vi "SO55 Create Monitor Task.vi"(2 "error in":errorcluster, 3 "Input":T1) -> (0 "error out":errorcluster, 1 "task out":refnum<k21>)   [LabVIEW 2012]
uses:
  <vilib>/DAQmx/create/channels.llb/DAQmx Create Channel (AI-Voltage-Basic).vi
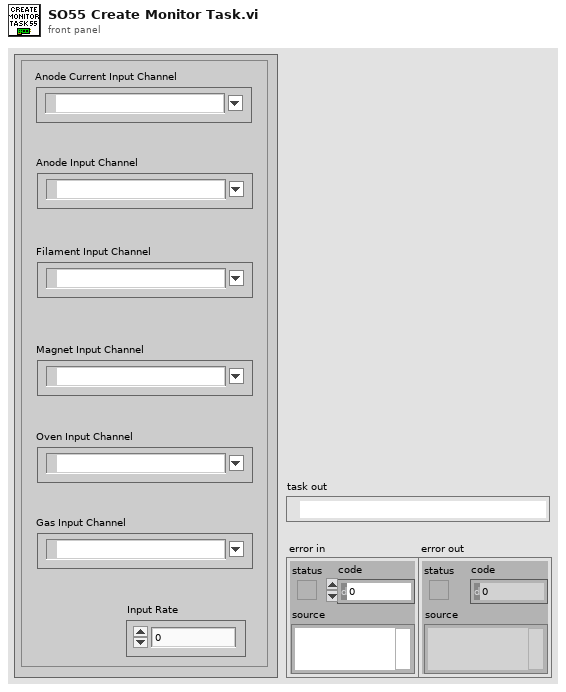
[diagram p1: front panel]
types:
  T1 = cluster{"Anode Input Channel":tag, "Filament Input Channel":tag, "Magnet Input Channel":tag, "Oven Input Channel":tag, "Gas Input Channel":tag, "Input Rate":dbl, "Anode Current Input Channel":tag}
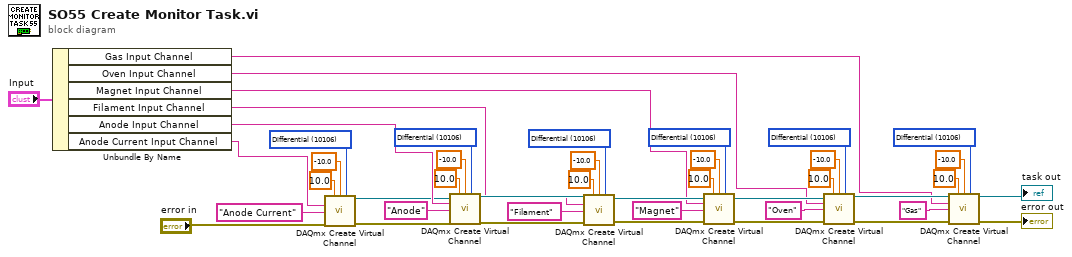
[diagram p0: block diagram]
diagram:
  w7 = 10106 items=["default"=-1, "RSE"=10083, "NRSE"=10078, "Differential"=10106, "Pseudodifferential"=12529] ("input terminal configuration")
  w19 = 10106 items=["default"=-1, "RSE"=10083, "NRSE"=10078, "Differential"=10106, "Pseudodifferential"=12529] ("input terminal configuration")
  w40 = 10106 items=["default"=-1, "RSE"=10083, "NRSE"=10078, "Differential"=10106, "Pseudodifferential"=12529] ("input terminal configuration")
  w34 = 10106 items=["default"=-1, "RSE"=10083, "NRSE"=10078, "Differential"=10106, "Pseudodifferential"=12529] ("input terminal configuration")
  w29 = 10106 items=["default"=-1, "RSE"=10083, "NRSE"=10078, "Differential"=10106, "Pseudodifferential"=12529] ("input terminal configuration")
  w24 = 10106 items=["default"=-1, "RSE"=10083, "NRSE"=10078, "Differential"=10106, "Pseudodifferential"=12529] ("input terminal configuration")
  n1 = Unbundle By Name("Input") -> ("Gas Input Channel"=w10:tag, "Oven Input Channel"=w11:tag, "Magnet Input Channel"=w12:tag, "Filament Input Channel"=w13:tag, "Anode Input Channel"=w14:tag, "Anode Current Input Channel"=w2:tag)
  n2 = call-poly <vilib>:"DAQmx Create Virtual Channel.vi"("maximum value"=10.0, "minimum value"=-10.0, "input terminal configuration"=w7, "physical channels"=w2, "name to assign"="Anode Current", "error in"="error in") -> ("task out"=w3:refnum<k21>, "error out"=w4:errorcluster)  [unwired: 8 in]
  n3 = call-poly <vilib>:"DAQmx Create Virtual Channel.vi"("task in"=w3, "maximum value"=10.0, "minimum value"=-10.0, "input terminal configuration"=w19, "physical channels"=w14, "name to assign"="Anode", "error in"=w4) -> ("task out"=w16:refnum<k21>, "error out"=w15:errorcluster)  [unwired: 7 in]
  n4 = call-poly <vilib>:"DAQmx Create Virtual Channel.vi"("task in"=w16, "maximum value"=10.0, "minimum value"=-10.0, "input terminal configuration"=w24, "physical channels"=w13, "name to assign"="Filament", "error in"=w15) -> ("task out"=w31:refnum<k21>, "error out"=w32:errorcluster)  [unwired: 7 in]
  n5 = call-poly <vilib>:"DAQmx Create Virtual Channel.vi"("task in"=w31, "maximum value"=10.0, "minimum value"=-10.0, "input terminal configuration"=w29, "physical channels"=w12, "name to assign"="Magnet", "error in"=w32) -> ("task out"=w43:refnum<k21>, "error out"=w37:errorcluster)  [unwired: 7 in]
  n6 = call-poly <vilib>:"DAQmx Create Virtual Channel.vi"("task in"=w43, "maximum value"=10.0, "minimum value"=-10.0, "input terminal configuration"=w34, "physical channels"=w11, "name to assign"="Oven", "error in"=w37) -> ("task out"=w44:refnum<k21>, "error out"=w42:errorcluster)  [unwired: 7 in]
  n7 = call-poly <vilib>:"DAQmx Create Virtual Channel.vi"("task in"=w44, "maximum value"=10.0, "minimum value"=-10.0, "input terminal configuration"=w40, "physical channels"=w10, "name to assign"="Gas", "error in"=w42) -> ("task out"=→"task out":refnum<k21>, "error out"=→"error out":errorcluster)  [unwired: 7 in]
